vi "EnqueueGUIMultipleUpdate.vi"(6 "FSContext":T1={"COMHandler"="", "HelloResponse"="", "FTDIDetected"=FALSE, "DeviceDetected"=FALSE, "TransferRefusedByUser"=FALSE, "AvailablePacketsNr"=0, "RequestType"=enum."NONE", "Response"="", "Packet(s)Available"=FALSE, "DownloadSuccess"=FALSE, "AppendDonwloadedPackets"=FALSE, "AppendLoadedPackets"=FALSE, "CfgDevWhenAvailable"=FALSE, "Packets"=[], "COMConfig"={"BaudRate"=9600, "DataBits"=8, "Parity"=enum."None", "StopBits"=10, "DataTransferTimeout[ms]"=10000, "FastTransferTimeout[ms]"=100, "ConnTries"=0, "MsWaitBeforeRetry"=0}, "ActivePacketID"=0, "AccelData"=[], "GyroData"=[], "ActiveMeasurementConfig"={"Frequency"=100, "Resolution[b]"=16, "AccelFSRange"=enum."+/-8g", "GyroFSRange"=enum."+/-1000dps"}, "OkayResponse"="", "MenuTags"={"SavePacketsTag"="", "ExportToCSVTag"="", "ExportToJSONTag"="", "ConfigureDeviceTag"="", "OpenPacketsTag"="", "OpenAndAppendPacketsTag"="", "EditCommentTag"="", "TakeGraphsScreenshotTag"=""}} {"ActiveMeasurementConfig"."Resolution[b]" min=4 max=16 step=1; "ActiveMeasurementConfig"."Frequency" min=1 max=10000000 step=1; "Packets"."MeasurementConfig"."Resolution[b]" min=4 max=16 step=1; "Packets"."MeasurementConfig"."Frequency" min=1 max=10000000 step=1; "COMConfig"."StopBits" items=["1.0"=10, "1.5"=15, "2.0"=20]; "COMConfig"."DataBits" min=7 max=9 step=1; "COMConfig"."BaudRate" min=9600 max=921600 step=1}, 8 "ErrorIn":errorcluster, 10 "GUIOperations":T11[](array[typedef]), 11 "Queue in":refnum<queue>) -> (0 "ErrorOut":errorcluster, 3 "QeueueOut":refnum<queue>)   [LabVIEW 2016]
doc: "This VI adds specific GUI operations for processing. It also requires FSContext in order to know what kind of values should be updated."
uses:
  QueueGUI/QueueGUIContext.ctl
  FSContext.ctl
  Requests/RequestType.ctl
  Packet.ctl
  Sample.ctl
  Reading.ctl
  MeasurementConfig.ctl
  Measurement/AccelFSRange.ctl
  Measurement/GyroFSRange.ctl
  FTDI/COMConfig.ctl
  MenuTags.ctl
  QueueGUI/GUIOperation.ctl
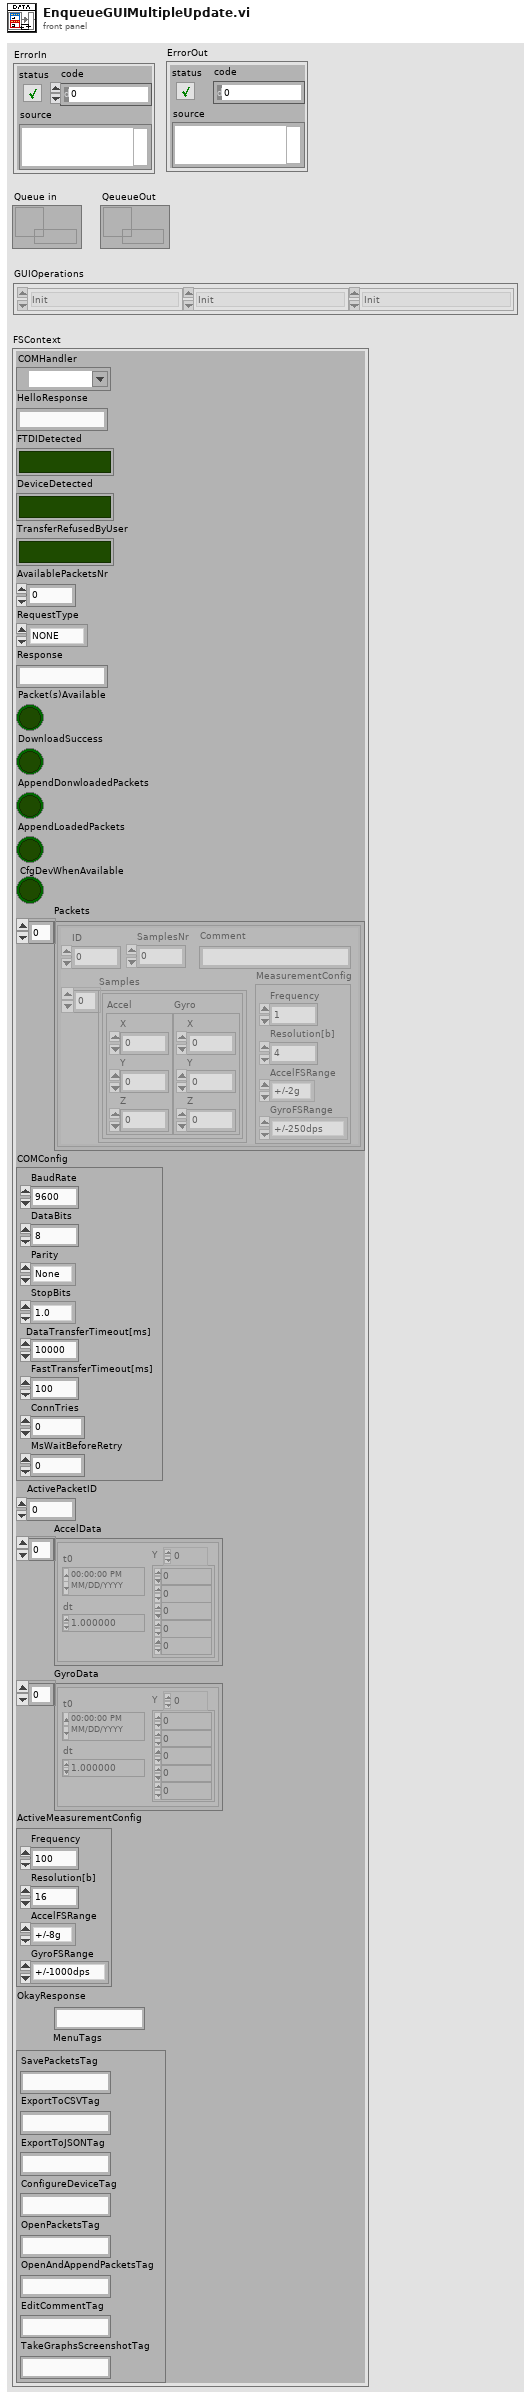
[diagram p1: front panel]
types:
  T1 = typedef "FSContext.ctl" = cluster{"COMHandler":refnum<visa-resource-name>, "HelloResponse":string, "FTDIDetected":bool, "DeviceDetected":bool, "TransferRefusedByUser":bool, "AvailablePacketsNr":u32, "RequestType":T2, "Response":string, "Packet(s)Available":bool, "DownloadSuccess":bool, "AppendDonwloadedPackets":bool, "AppendLoadedPackets":bool, "CfgDevWhenAvailable":bool, "Packets":T3[], "COMConfig":T9, "ActivePacketID":i32, "AccelData":waveform(dbl)[], "GyroData":waveform(dbl)[], "ActiveMeasurementConfig":T6, "OkayResponse":string, "MenuTags":T10}
  T2 = typedef "RequestType.ctl" = enum16{"NONE", "Reset", "Hello", "GetPacketsNr", "GetPacket", "GetConfig", "SetConfig", "SendConfig", "Goodbye"}
  T3 = typedef "Packet.ctl" = cluster{"ID":u32, "SamplesNr":u32, "Samples":T4[], "MeasurementConfig":T6, "Comment":string}
  T4 = typedef "Sample.ctl" = cluster{"Accel":T5, "Gyro":T5}
  T5 = typedef "Reading.ctl" = cluster{"X":i16, "Y":i16, "Z":i16}
  T6 = typedef "MeasurementConfig.ctl" = cluster{"Frequency":u32, "Resolution[b]":u32, "AccelFSRange":T7, "GyroFSRange":T8}
  T7 = typedef "AccelFSRange.ctl" = enum16{"+/-2g", "+/-4g", "+/-8g", "+/-16g"}
  T8 = typedef "GyroFSRange.ctl" = enum16{"+/-250dps", "+/-500dps", "+/-1000dps", "+/-2000dps"}
  T9 = typedef "COMConfig.ctl" = cluster{"BaudRate":u32, "DataBits":u16, "Parity":enum16{"None", "Odd", "Even", "Mark", "Space"}, "StopBits":u16, "DataTransferTimeout[ms]":u32, "FastTransferTimeout[ms]":u32, "ConnTries":i32, "MsWaitBeforeRetry":u32}
  T10 = typedef "MenuTags.ctl" = cluster{"SavePacketsTag":string, "ExportToCSVTag":string, "ExportToJSONTag":string, "ConfigureDeviceTag":string, "OpenPacketsTag":string, "OpenAndAppendPacketsTag":string, "EditCommentTag":string, "TakeGraphsScreenshotTag":string}
  T11 = typedef "GUIOperation.ctl" = enum16{"NONE", "Init", "UpdateSerialContext", "UpdateResponse", "UpdateFlags", "UpdateNumerics", "UpdatePacketList", "DisplayPacket", "ResetPacketSelectionFlags", "StopGUI"}
  T12 = typedef "QueueGUIContext.ctl" = cluster{"Content":T1, "GUIOperation":T11}
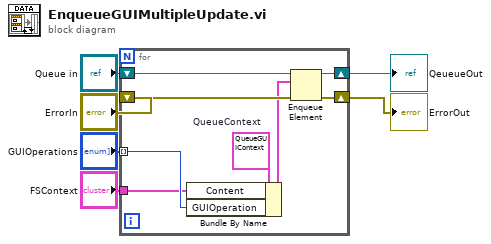
[diagram p0: block diagram]
diagram:
  n1 = for {
    shift-right: [w14] -> w6
    shift-left: "ErrorIn" -> [w12]
    shift-right: [w13] -> w5
    shift-left: "Queue in" -> [w11]
    tunnel: "GUIOperations" -> [w8] mode=indexing
    tunnel: "FSContext" -> [w7]
    w9 = T12 {"Content"={"COMHandler"="", "HelloResponse"="", "FTDIDetected"=FALSE, "DeviceDetected"=FALSE, "TransferRefusedByUser"=FALSE, "AvailablePacketsNr"=0, "RequestType"=enum."NONE", "Response"="", "Packet(s)Available"=FALSE, "DownloadSuccess"=FALSE, "AppendDonwloadedPackets"=FALSE, "AppendLoadedPackets"=FALSE, "CfgDevWhenAvailable"=FALSE, "Packets"=[], "COMConfig"={"BaudRate"=9600, "DataBits"=8, "Parity"=enum."None", "StopBits"=10, "DataTransferTimeout[ms]"=10000, "FastTransferTimeout[ms]"=100, "ConnTries"=0, "MsWaitBeforeRetry"=0}, "ActivePacketID"=0, "AccelData"=[], "GyroData"=[], "ActiveMeasurementConfig"={"Frequency"=100, "Resolution[b]"=16, "AccelFSRange"=enum."+/-8g", "GyroFSRange"=enum."+/-1000dps"}, "OkayResponse"="", "MenuTags"={"SavePacketsTag"="", "ExportToCSVTag"="", "ExportToJSONTag"="", "ConfigureDeviceTag"="", "OpenPacketsTag"="", "OpenAndAppendPacketsTag"="", "EditCommentTag"="", "TakeGraphsScreenshotTag"=""}}, "GUIOperation"=enum."Init"}  # QueueContext
    n2 = Bundle By Name(cluster=w9, "Content"=w7, "GUIOperation"=w8) -> (w10:T12)
    n3 = Enqueue Element(queue=w11, element=w10, error in (no error)=w12) -> (queue out=w13:refnum<queue>, error out=w14:errorcluster)  [unwired: 1 in, 1 out]
  }
  "ErrorOut" <- w6
  "QeueueOut" <- w5
